vi "SubPanel Host-Core_Process.vi"(0 "FTW Actor Instance Configuration":string="{\n  \"Identity\": \"SubPanel Host\",\n  \"InboxAddress\": \"inproc://*\",\n  \"PublisherAddress\": \"\",\n  \"LoggerAddress\": \"\",\n  \"DebugEnableInboxLogging\": false,\n  \"DebugEnableJobLogging\": false,\n  \"LauncherAddress\": \"\"\n}") -> (15 "Error":errorcluster)   [LabVIEW 2013, in "SubPanel Host-Core.lvclass"]
uses:
  SubPanel Host-Core.lvclass
  source/actor/Message/Base/FTW-Message.lvclass
  SubPanel Host-Core.lvclass/SubPanel Host-Core.ctl
  SubPanel Guest/SubPanel Guest.lvclass
  source/actor/Instance/FTW-ActorInstance.lvclass/FTW-ActorInstance.ctl
  source/actor/JobSequencer/FTW-SEQ-Current.vi
  source/actor/Instance/FTW-ActorInstance.lvclass
  source/actor/Message/Request/FTW-Message-IncomingRequest.lvclass
  source/actor/Ether/FTW-Ether.lvclass
panel:
  in  "Close":bool
  in  "Open":bool
  # "Inputs"
  # "Outputs"
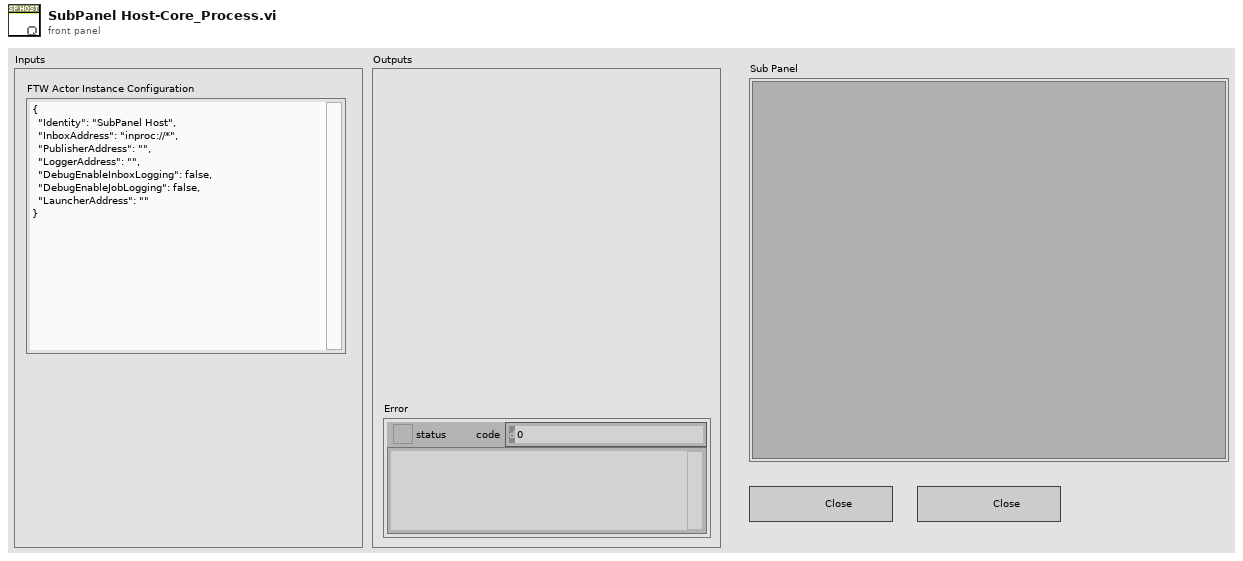
[diagram p1: front panel]
types:
  T1 = cluster{"Incoming Requests":refnum<event-registration>, "Local Messages":refnum<event-registration>, "Additional Registration Types":refnum<event-registration>}
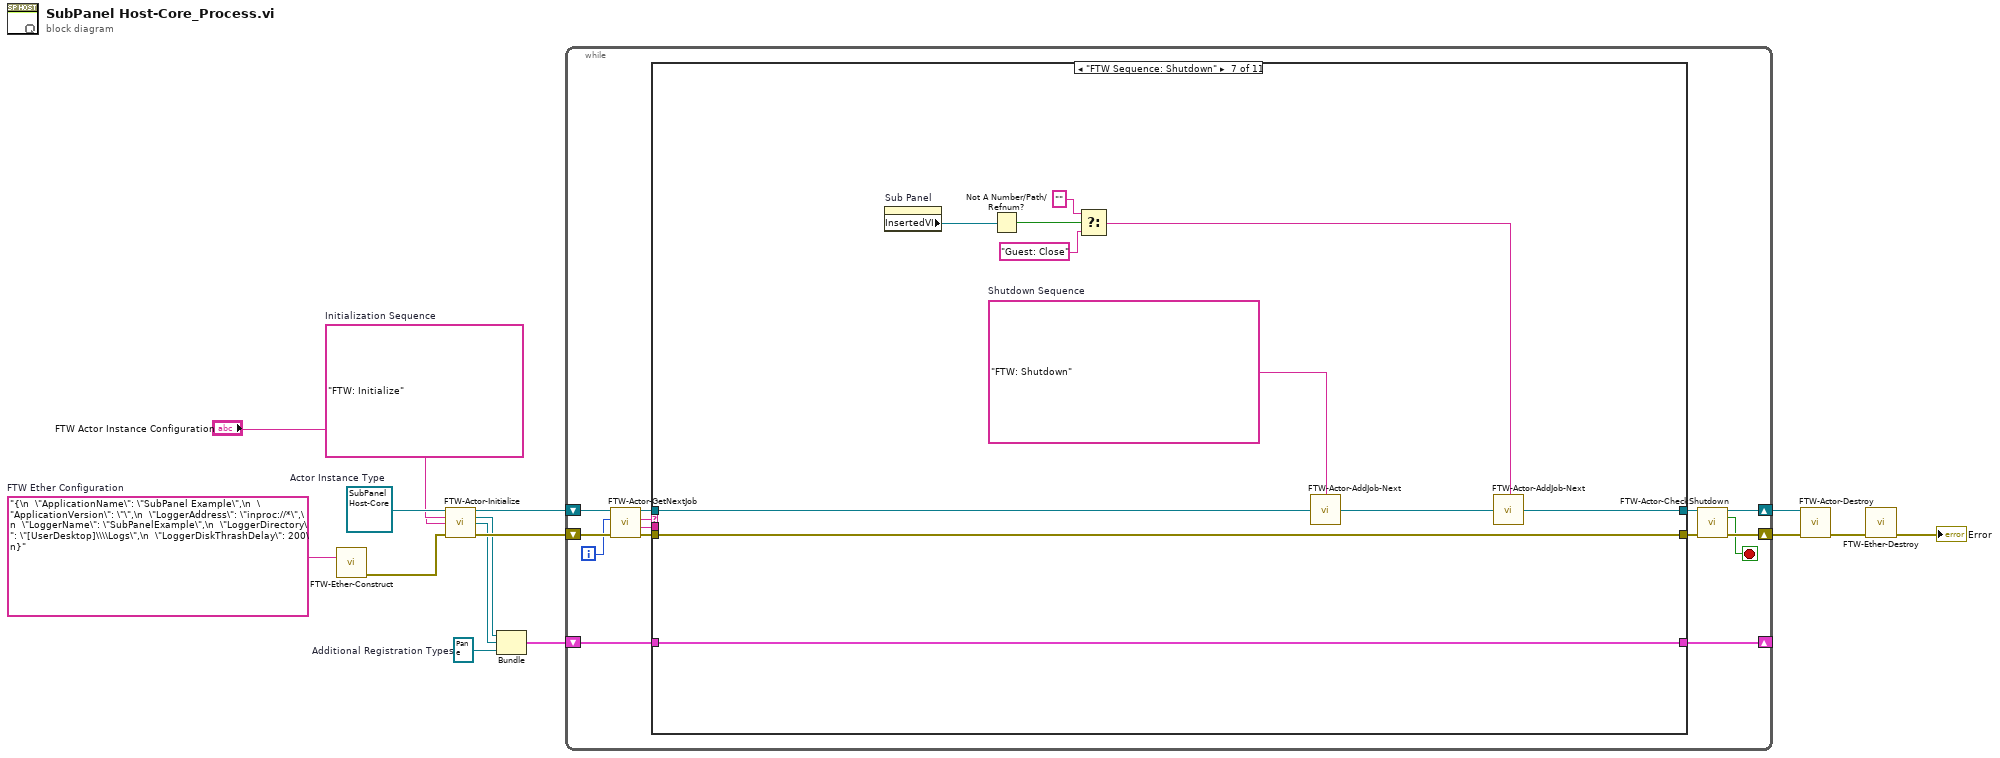
[diagram p0: block diagram]
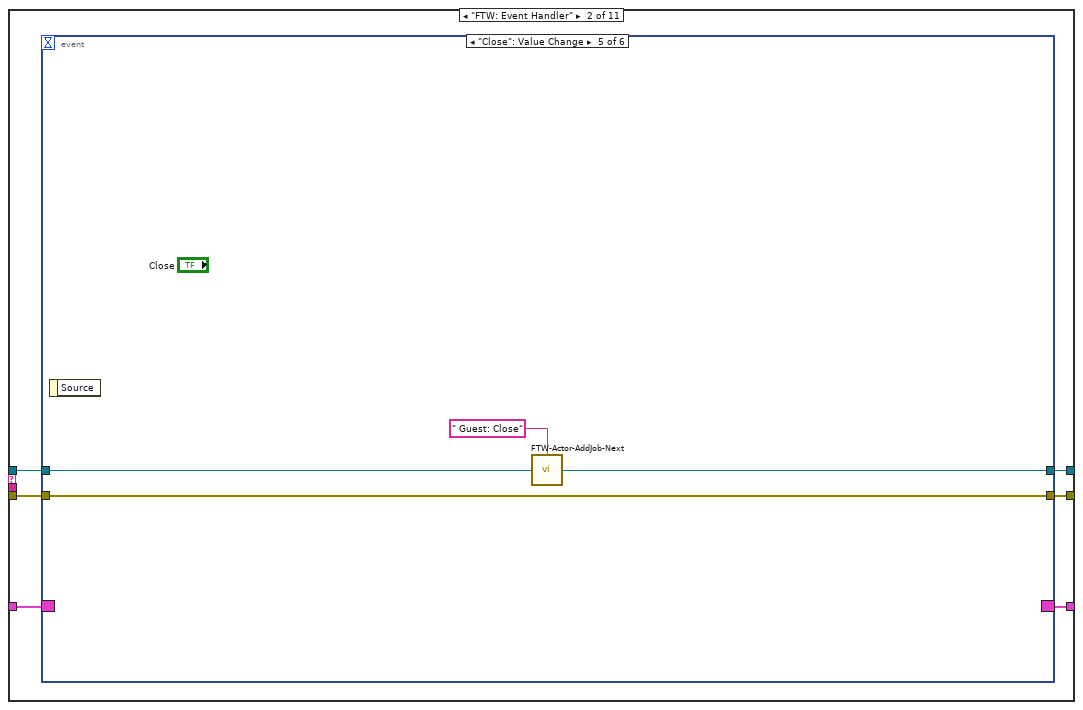
[diagram p3: hidden frame]
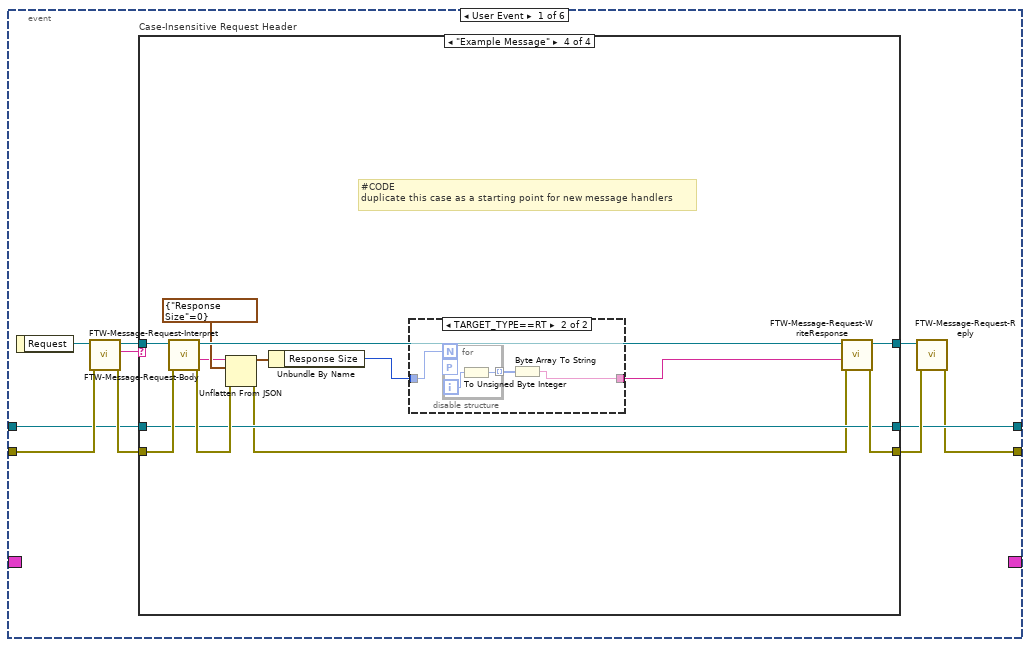
[diagram p4: hidden frame]
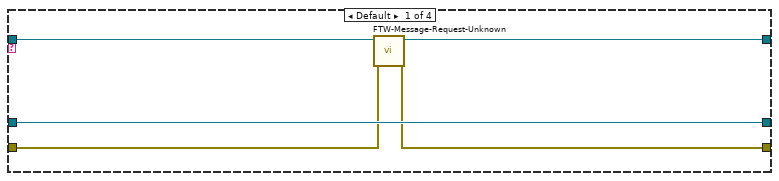
[diagram p5: hidden frame]
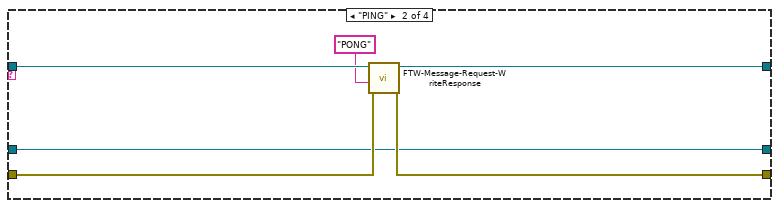
[diagram p6: hidden frame]
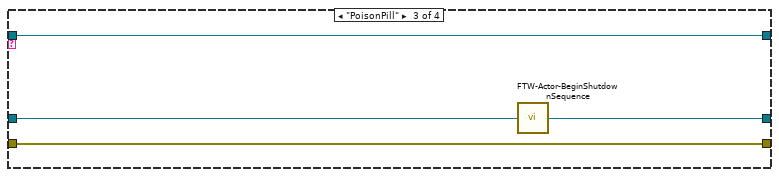
[diagram p7: hidden frame]
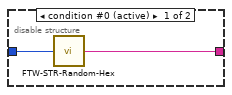
[diagram p8: hidden frame]
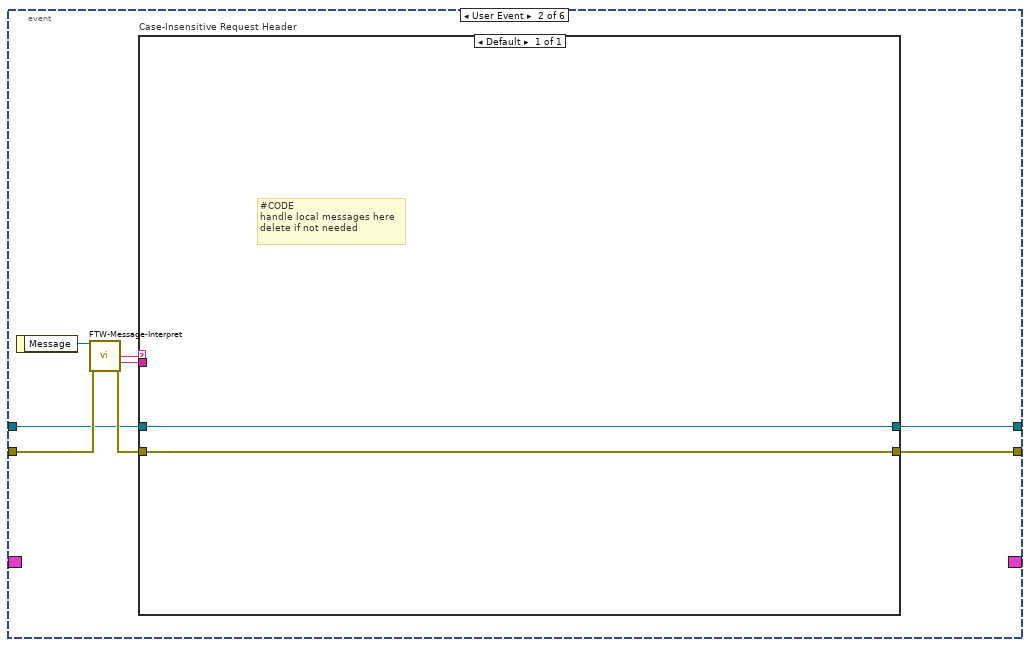
[diagram p9: hidden frame]
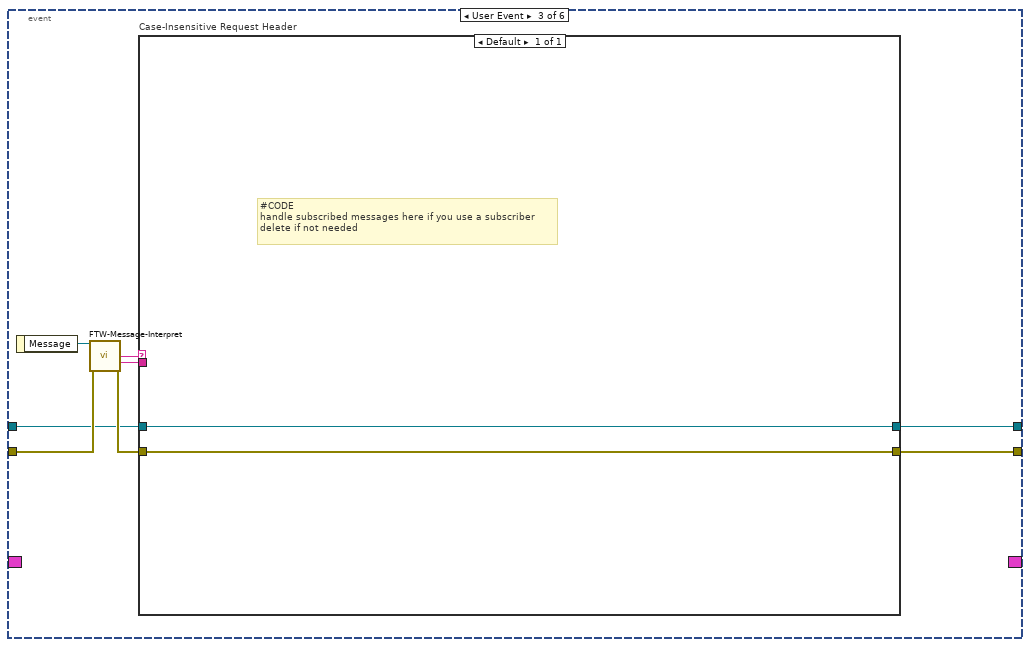
[diagram p10: hidden frame]
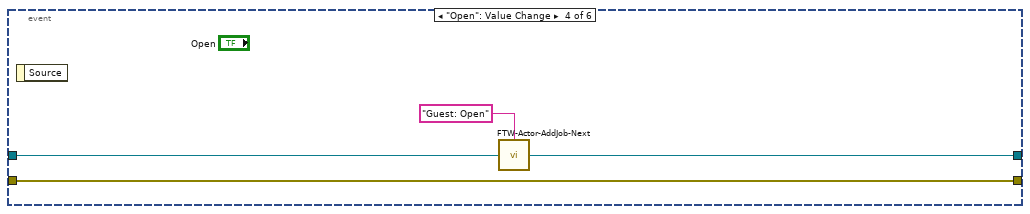
[diagram p11: hidden frame]
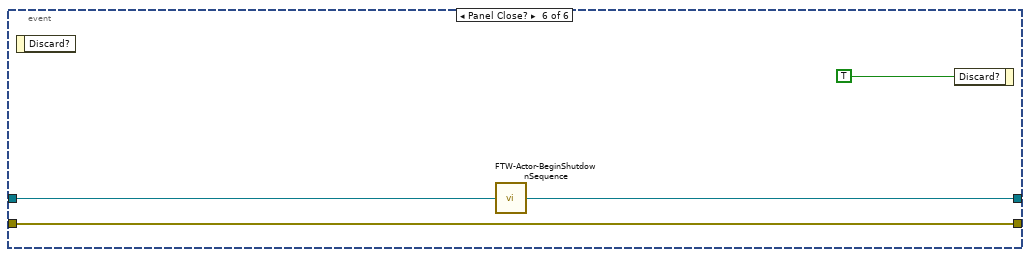
[diagram p12: hidden frame]
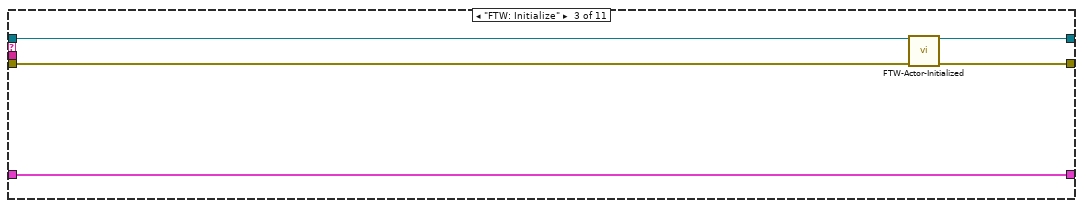
[diagram p13: hidden frame]
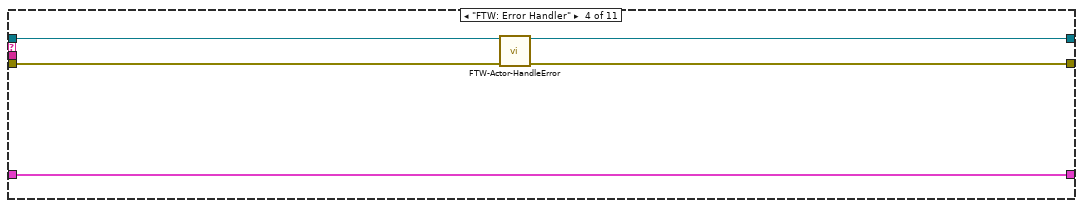
[diagram p14: hidden frame]
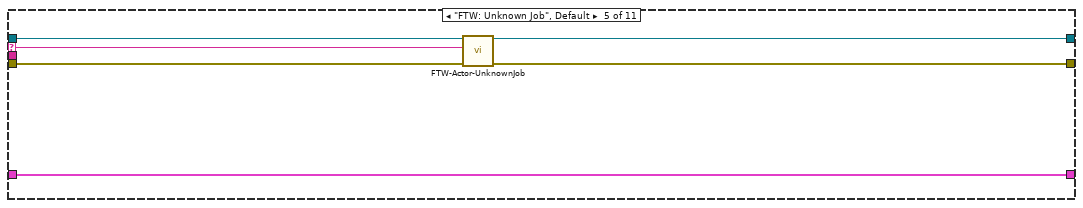
[diagram p15: hidden frame]
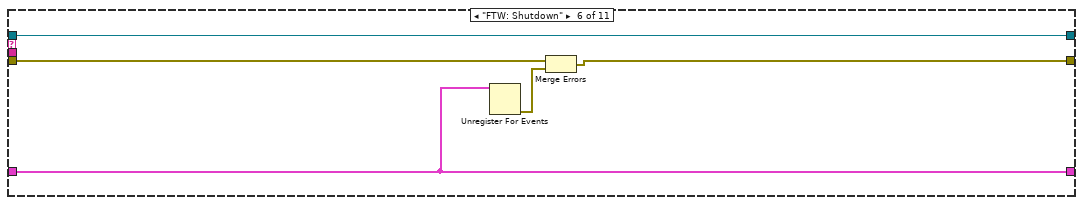
[diagram p16: hidden frame]
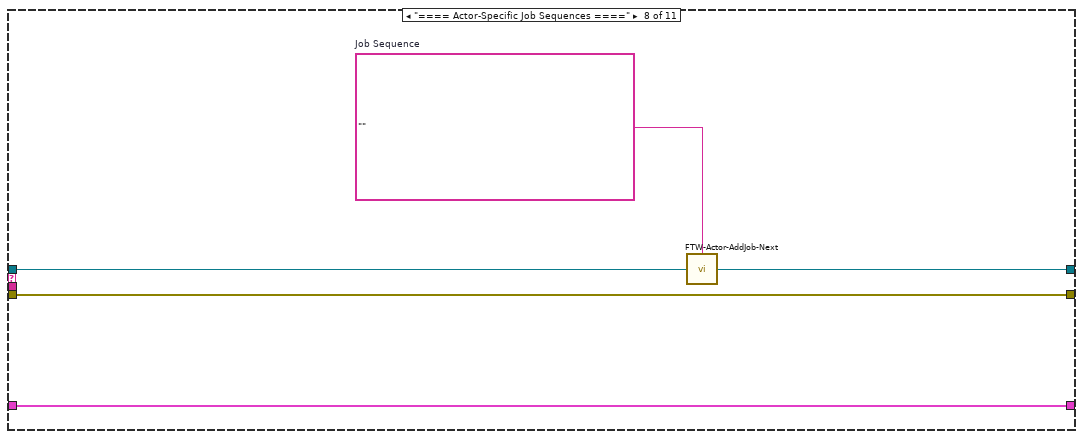
[diagram p17: hidden frame]
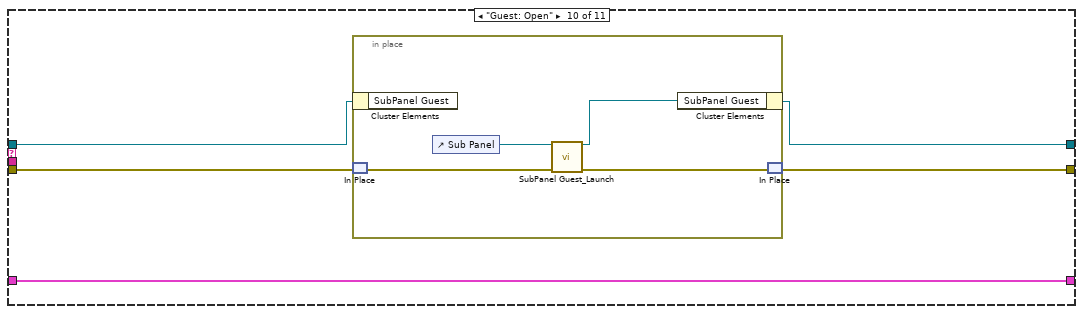
[diagram p19: hidden frame]
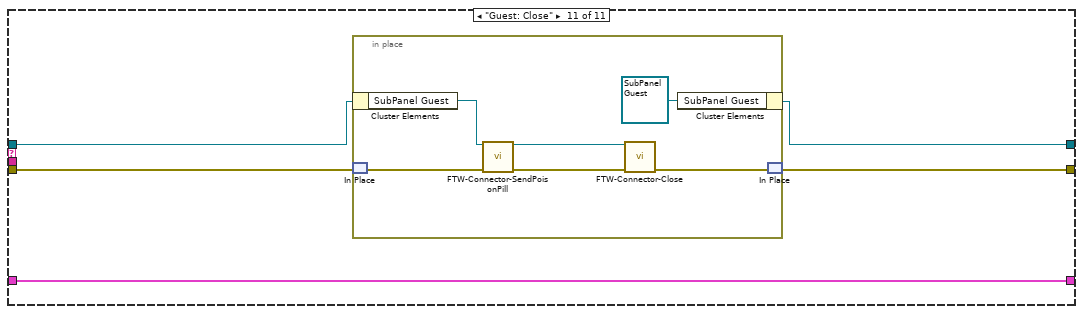
[diagram p20: hidden frame]
diagram:
  w3 = "{\n  \"ApplicationName\": \"SubPanel Example\",\n  \"ApplicationVersion\": \"\",\n  \"LoggerAddress\": \"inproc://*\",\n  \"LoggerName\": \"SubPanelExample\",\n  \"LoggerDirectory\": \"[UserDesktop]\\\\Logs\",\n  \"LoggerDiskThrashDelay\": 200\n}"  # FTW Ether Configuration
  w5 = refnum<event-registration> refnum  # Additional Registration Types
  w11 = refnum<class "SubPanel Host-Core.lvclass"> refnum  # Actor Instance Type
  w10 = "FTW: Initialize"  # Initialization Sequence
  n1 = call "FTW-Ether-Construct.vi"("FTW Ether Configuration"=w3) -> ("error out"=w2:errorcluster)  [unwired: 14 in]
  n2 = call-dynamic "FTW-Actor-Initialize.vi"("FTW Actor Instance Type"=w11, "Initialization Job Sequence"=w10, "Actor Instance Configuration"="FTW Actor Instance Configuration", "error in"=w2) -> ("FTW Actor Instance"=w4:refnum<class "SubPanel Host-Core.lvclass">, "Incoming Requests"=w7:refnum<event-registration>, "Local Messages"=w6:refnum<event-registration>, "error out"=w12:errorcluster)  [unwired: 8 in]
  n3 = Bundle("Incoming Requests"=w7, "Local Messages"=w6, "Additional Registration Types"=w5) -> (w9:T1)  [unwired: 1 in]
  n4 = while {
    shift-right: [w19] -> w14
    shift-left: w12 -> [w26]
    shift-right: [w16] -> _
    shift-left: w9 -> [w29]
    shift-right: [w21] -> w15
    shift-left: w4 -> [w28]
    i -> [w17]
    stop <- w18 stop-if-true
    n5 = call "FTW-Actor-GetNextJob.vi"("error in"=w26, "Jobs Performed"=w17, "FTW Actor Instance"=w28) -> ("error out"=w25:errorcluster, "Job Data"=w23:string, "Job Name"=w24:string, "FTW Actor Instance out"=w27:refnum<class "SubPanel Host-Core.lvclass">)  [unwired: 5 in]
    n6 = case shown="\"FTW Sequence: Shutdown\"" w24 {
      selector: w24 -> [_ _ _ _ w126 _ _ _ _ _ _]
      tunnel: [w31 w38 w116 w121 w129 w135 w146 w151 w155 w157 w166] -> w20
      tunnel: w25 -> [w31 w37 w119 w123 w130 w136 w146 w151 w155 w158 w167]
      tunnel: w29 -> [w32 w33 w120 w125 w131 w132 w147 w152 w154 w160 w169]
      tunnel: [w32 w36 w120 w125 w131 w132 w147 w152 w154 w160 w169] -> w16
      tunnel: w23 -> [_ _ _ _ _ _ _ _ _ _ _]
      tunnel: [w30 w35 w117 w122 w127 w133 w142 w149 w153 w156 w165] -> w22
      tunnel: w27 -> [w30 w34 w118 w124 w128 w133 w145 w150 w153 w159 w168]
      frame "==== Featherweight Framework Jobs ====" {
      }
      frame "FTW: Event Handler" {
        n7 = event shown="[4] \"Close\": Value Change" {
          selector: w33 -> [_ _ _ _ _ _]
          dyn-events: [_ _ _ _ _ _] -> w36
          timeout: _ -> [_ _ _ _ _ _]
          tunnel: [w40 w88 w98 w107 w111 w114] -> w38
          tunnel: w37 -> [w46 w89 w99 w107 w111 w114]
          tunnel: [w44 w87 w97 w105 w109 w112] -> w35
          tunnel: w34 -> [w43 w86 w96 w106 w110 w113]
          event User Event {
            n8 = event-data() -> ("Request"=w47:refnum<class "FTW-Message-IncomingRequest.lvclass">)  [unwired: 1 in]
            n9 = call "FTW-Message-Request-Interpret.vi"("error in"=w46, "FTW Incoming Request"=w47) -> ("error out"=w48:errorcluster, "Request Header"=w42:string, "FTW Incoming Request out"=w41:refnum<class "FTW-Message-IncomingRequest.lvclass">)  [unwired: 7 in]
            n10 = case "Case-Insensitive Request Header" shown="\"Example Message\"" w42 {
              tunnel: [w51 w57 w62 w73] -> w45
              tunnel: w48 -> [w52 w58 w62 w76]
              tunnel: [w53 w56 w63 w70] -> w44
              tunnel: w43 -> [w53 w56 w61 w70]
              tunnel: w41 -> [w50 w59 w60 w74]
              tunnel: [w49 w55 w60 w71] -> w39
              frame Default {
                n11 = call "FTW-Message-Request-Unknown.vi"("error in"=w52, "FTW Incoming Request"=w50) -> ("error out"=w51:errorcluster, "FTW Incoming Request Out"=w49:refnum<class "FTW-Message-IncomingRequest.lvclass">)  [unwired: 8 in]
              }
              frame "PING" {
                n12 = call "FTW-Message-Request-WriteResponse.vi"("error in"=w58, "Response Body"="PONG" ("Response Header"), "FTW Incoming Request"=w59) -> ("error out"=w57:errorcluster, "FTW Incoming Request out"=w55:refnum<class "FTW-Message-IncomingRequest.lvclass">)  [unwired: 7 in]
              }
              frame "PoisonPill" {
                n13 = call "FTW-Actor-BeginShutdownSequence.vi"("FTW Actor Instance"=w61) -> ("FTW Actor Instance out"=w63:refnum<class "SubPanel Host-Core.lvclass">)  [unwired: 3 in]
              }
              frame "Example Message" {
                # "#CODE\nduplicate this case as a starting point for new message handlers"
                n14 = call "FTW-Message-Request-Body.vi"("error in"=w76, "FTW Incoming Request"=w74) -> ("error out"=w75:errorcluster, "Request Body"=w67:string, "FTW Incoming Request out"=w72:refnum<class "FTW-Message-IncomingRequest.lvclass">)  [unwired: 7 in]
                n15 = Unflatten From JSON(JSON string=w67, type and defaults=cluster{"Response Size":i32} {"Response Size"=0}, error in (no error)=w75) -> (value=w66:cluster{"Response Size":i32}, error out=w69:errorcluster)  [unwired: 4 in]
                n16 = Unbundle By Name(w66) -> ("Response Size"=w65:i32)
                n17 = disable-structure shown="TARGET_TYPE==RT" {
                  disable-tunnel: w65 -> [w78 w81]
                  disable-tunnel: [w77 w79] -> w64
                  frame condition #0 (active) {
                    n18 = call "FTW-STR-Random-Hex.vi"("String Length"=w78) -> ("Random Hex String"=w77:string)  [unwired: 3 in]
                  }
                  frame condition #1 {
                    n19 = for {
                      N: w81 -> [_]
                      workers-P: _ -> [_]
                      tunnel: [w82] -> w80 mode=indexing
                      i -> [w83]
                      n20 = To Unsigned Byte Integer(number=w83) -> (unsigned 8bit integer=w82:u8)
                    }
                    n21 = Byte Array To String(unsigned byte array=w80) -> (string=w79:string)
                  }
                }
                n22 = call "FTW-Message-Request-WriteResponse.vi"("error in"=w69, "Response Body"=w64, "FTW Incoming Request"=w72) -> ("error out"=w73:errorcluster, "FTW Incoming Request out"=w71:refnum<class "FTW-Message-IncomingRequest.lvclass">)  [unwired: 7 in]
              }
            }
            n23 = call "FTW-Message-Request-Reply.vi"("error in"=w45, "FTW Incoming Request"=w39) -> ("error out"=w40:errorcluster)  [unwired: 8 in, 1 out]
          }
          event User Event {
            n24 = event-data() -> ("Message"=w90:refnum<class "FTW-Message.lvclass">)  [unwired: 1 in]
            n25 = call-dynamic "FTW-Message-Interpret.vi"("FTW Message"=w90, "error in"=w89) -> ("Message Header"=w84:string, "Message Body"=w85:string, "error out"=w91:errorcluster)  [unwired: 9 in, 2 out]
            n26 = case "Case-Insensitive Request Header" shown="Default" w84 {
              tunnel: [w92] -> w88
              tunnel: w91 -> [w92]
              tunnel: [w93] -> w87
              tunnel: w86 -> [w93]
              tunnel: w85 -> [_]
              frame Default {
                # "#CODE\nhandle local messages here\ndelete if not needed"
              }
            }
          }
          event User Event {
            n27 = event-data() -> ("Message"=w100:refnum<class "FTW-Message.lvclass">)  [unwired: 1 in]
            n28 = call-dynamic "FTW-Message-Interpret.vi"("FTW Message"=w100, "error in"=w99) -> ("Message Header"=w94:string, "Message Body"=w95:string, "error out"=w101:errorcluster)  [unwired: 9 in, 2 out]
            n29 = case "Case-Insensitive Request Header" shown="Default" w94 {
              tunnel: [w102] -> w98
              tunnel: w101 -> [w102]
              tunnel: [w103] -> w97
              tunnel: w96 -> [w103]
              tunnel: w95 -> [_]
              frame Default {
                # "#CODE\nhandle subscribed messages here if you use a subscriber\ndelete if not needed"
              }
            }
          }
          event "Open": Value Change {
            n30 = event-data() -> ()  [unwired: 1 in, 1 out]
            n31 = call "FTW-Actor-AddJob-Next.vi"("Add Next in Job Queue"="Guest: Open", "FTW Actor Instance"=w106) -> ("FTW Actor Instance out"=w105:refnum<class "SubPanel Host-Core.lvclass">)  [unwired: 2 in]
          }
          event "Close": Value Change {
            n32 = event-data() -> ()  [unwired: 1 in, 1 out]
            n33 = call "FTW-Actor-AddJob-Next.vi"("Add Next in Job Queue"=" Guest: Close", "FTW Actor Instance"=w110) -> ("FTW Actor Instance out"=w109:refnum<class "SubPanel Host-Core.lvclass">)  [unwired: 2 in]
          }
          event Panel Close? {
            n34 = event-data() -> ()  [unwired: 1 in, 1 out]
            n35 = call "FTW-Actor-BeginShutdownSequence.vi"("FTW Actor Instance"=w113) -> ("FTW Actor Instance out"=w112:refnum<class "SubPanel Host-Core.lvclass">)  [unwired: 3 in]
            n36 = event-data("Discard?"=TRUE) -> ()  [unwired: 1 in, 1 out]
          }
        }
      }
      frame "FTW: Initialize" {
        n37 = call-dynamic "FTW-Actor-Initialized.vi"("FTW Actor Instance"=w118, "error in"=w119) -> ("FTW Actor Instance out"=w117:refnum<class "SubPanel Host-Core.lvclass">, "error out"=w116:errorcluster)  [unwired: 12 in]
      }
      frame "FTW: Error Handler" {
        n38 = call-dynamic "FTW-Actor-HandleError.vi"("FTW Actor Instance"=w124, "error in"=w123) -> ("FTW Actor Instance out"=w122:refnum<class "SubPanel Host-Core.lvclass">, "error out"=w121:errorcluster)  [unwired: 11 in, 1 out]
      }
      frame "FTW: Unknown Job", Default {
        n39 = call-dynamic "FTW-Actor-UnknownJob.vi"("FTW Actor Instance"=w128, "Unknown Job"=w126, "error in"=w130) -> ("FTW Actor Instance out"=w127:refnum<class "SubPanel Host-Core.lvclass">, "error out"=w129:errorcluster)  [unwired: 11 in]
      }
      frame "FTW: Shutdown" {
        n40 = Unregister For Events(event registration refnum=w132) -> (error out=w134:errorcluster)  [unwired: 1 in]
        n41 = Merge Errors(w136, w134) -> (w135:errorcluster)
      }
      frame "FTW Sequence: Shutdown" {
        w143 = "FTW: Shutdown"  # Shutdown Sequence
        n42 = property on="Sub Panel" class="SubPnl"() -> ("InsertedVI"=w141:refnum<vi>)  [unwired: 2 in, 2 out]
        n43 = Not A Number/Path/Refnum?(number/path/refnum=w141) -> (NaN/Path/Refnum?=w140:bool)
        n44 = Select(t="", s=w140, f="Guest: Close") -> (s? t:f=w139:string)
        n45 = call "FTW-Actor-AddJob-Next.vi"("Add Next in Job Queue"=w143, "FTW Actor Instance"=w145) -> ("FTW Actor Instance out"=w144:refnum<class "SubPanel Host-Core.lvclass">)  [unwired: 2 in]
        n46 = call "FTW-Actor-AddJob-Next.vi"("Add Next in Job Queue"=w139, "FTW Actor Instance"=w144) -> ("FTW Actor Instance out"=w142:refnum<class "SubPanel Host-Core.lvclass">)  [unwired: 2 in]
      }
      frame "==== Actor-Specific Job Sequences ====" {
        w148 = ""  # Job Sequence
        n47 = call "FTW-Actor-AddJob-Next.vi"("Add Next in Job Queue"=w148, "FTW Actor Instance"=w150) -> ("FTW Actor Instance out"=w149:refnum<class "SubPanel Host-Core.lvclass">)  [unwired: 2 in]
      }
      frame "==== Actor-Specific Jobs ====" {
      }
      frame "Guest: Open" {
        n48 = in-place {
          n49 = in-place-cluster #1(w159) -> ()  [unwired: 1 out]
          n50 = in-place-match #2(w158) -> (w164:errorcluster)
          n51 = control-ref of="Sub Panel"() -> (w162:refnum<vi>)
          n52 = call "SubPanel Guest_Launch.vi"("SubPanel"=w162, "error in"=w164) -> ("FTW Actor Connector"=w161:refnum<class "SubPanel Guest.lvclass">, "error out"=w163:errorcluster)  [unwired: 10 in, 2 out]
          n53 = in-place-cluster #1("SubPanel Guest"=w161) -> (w156:refnum<class "SubPanel Host-Core.lvclass">)
          n54 = in-place-match #2(w163) -> (w157:errorcluster)
        }
      }
      frame "Guest: Close" {
        n55 = in-place {
          n56 = in-place-cluster #3(w168) -> ("SubPanel Guest"=w173:refnum<class "SubPanel Guest.lvclass">)
          n57 = in-place-match #4(w167) -> (w175:errorcluster)
          n58 = call-dynamic "FTW-Connector-SendPoisonPill.vi"("FTW Actor Connector"=w173, "error in"=w175) -> ("FTW Actor Connector out"=w171:refnum<class "SubPanel Guest.lvclass">, "error out"=w174:errorcluster)  [unwired: 9 in, 3 out]
          n59 = call-dynamic "FTW-Connector-Close.vi"("FTW Actor Connector"=w171, "error in"=w174) -> ("error out"=w172:errorcluster)  [unwired: 13 in]
          n60 = in-place-cluster #3("SubPanel Guest"=refnum<class "SubPanel Guest.lvclass"> refnum) -> (w165:refnum<class "SubPanel Host-Core.lvclass">)
          n61 = in-place-match #4(w172) -> (w166:errorcluster)
        }
      }
    }
    n62 = call "FTW-Actor-CheckShutdown.vi"("FTW Actor Instance"=w22, "error in"=w20) -> ("FTW Actor Instance out"=w21:refnum<class "SubPanel Host-Core.lvclass">, "Shutdown?"=w18:bool, "error out"=w19:errorcluster)  [unwired: 11 in]
  }
  n63 = call-dynamic "FTW-Actor-Destroy.vi"("FTW Actor Instance"=w15, "error in"=w14) -> ("error out"=w13:errorcluster)  [unwired: 13 in]
  n64 = call "FTW-Ether-Destroy.vi"("error in"=w13) -> ("error out"=→"Error":errorcluster)  [unwired: 14 in]
